vi "SEM shutter.vi"(6 "Shutter close":bool, 7 "delay (ms)":u32=1000, 8 "Shutter AO4":tag="Log/ao3", 9 "Shutter AO3":tag="Log/ao2", 10 "Shutter AO2":tag="Log/ao1", 11 "Shutter AO1":tag="Log/ao0") -> (0 "error out":errorcluster)   [LabVIEW 2018]
uses:
  <vilib>/DAQmx/write.llb/DAQmx Write (Analog 1D DBL NChan 1Samp).vi
  <vilib>/DAQmx/create/channels.llb/DAQmx Create Channel (AO-Voltage-Basic).vi
  <vilib>/DAQmx/miscellaneous.llb/DAQmx Fill In Error Info.vi
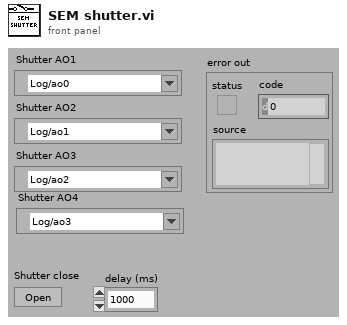
[diagram p1: front panel]
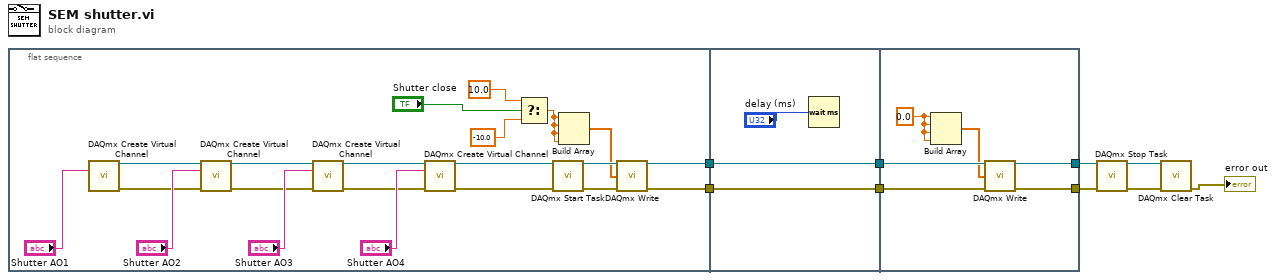
[diagram p0: block diagram]
diagram:
  n1 = flat-sequence {
    tunnel: [w28] -> w4
    tunnel: [w27] -> w2
    tunnel: w4 -> [w33]
    tunnel: [w33] -> w3
    tunnel: w2 -> [w32]
    tunnel: [w32] -> w1
    tunnel: [w36] -> w8
    tunnel: [w38] -> w9
    tunnel: w3 -> [w39]
    tunnel: w1 -> [w37]
    frame #0 {
      n2 = call-poly <vilib>:"DAQmx Create Virtual Channel.vi"("physical channels"="Shutter AO1") -> ("task out"=w20:refnum<k21>, "error out"=w19:errorcluster)  [unwired: 13 in]
      n3 = call-poly <vilib>:"DAQmx Create Virtual Channel.vi"("task in"=w20, "physical channels"="Shutter AO2", "error in"=w19) -> ("task out"=w12:refnum<k21>, "error out"=w11:errorcluster)  [unwired: 11 in]
      n4 = call-poly <vilib>:"DAQmx Create Virtual Channel.vi"("task in"=w12, "physical channels"="Shutter AO3", "error in"=w11) -> ("task out"=w14:refnum<k21>, "error out"=w13:errorcluster)  [unwired: 11 in]
      n5 = call-poly <vilib>:"DAQmx Create Virtual Channel.vi"("task in"=w14, "physical channels"="Shutter AO4", "error in"=w13) -> ("task out"=w16:refnum<k21>, "error out"=w15:errorcluster)  [unwired: 11 in]
      n6 = Select(t=10.0, s="Shutter close", f=-10.0) -> (s? t:f=w10:dbl)
      n7 = call <vilib>:"DAQmx Start Task.vi"("task/channels in"=w16, "error in"=w15) -> ("task out"=w30:refnum<k21>, "error out"=w29:errorcluster)  [unwired: 12 in]
      n8 = Build Array(w10, w10, w10, w10) -> (w22:dbl[])
      n9 = call-poly <vilib>:"DAQmx Write.vi"("task/channels in"=w30, "data"=w22, "error in"=w29) -> ("task out"=w28:refnum<k21>, "error out"=w27:errorcluster)  [unwired: 10 in, 1 out]
    }
    frame #1 {
      n10 = Wait (ms)(milliseconds to wait="delay (ms)") -> ()  [unwired: 1 out]
    }
    frame #2 {
      w34 = 0.0 ("element")
      n11 = Build Array(w34, w34, w34, w34) -> (w35:dbl[])
      n12 = call-poly <vilib>:"DAQmx Write.vi"("task/channels in"=w39, "data"=w35, "error in"=w37) -> ("task out"=w38:refnum<k21>, "error out"=w36:errorcluster)  [unwired: 10 in, 1 out]
    }
  }
  n13 = call <vilib>:"DAQmx Stop Task.vi"("task/channels in"=w9, "error in"=w8) -> ("task out"=w6:refnum<k21>, "error out"=w7:errorcluster)  [unwired: 12 in]
  n14 = call <vilib>:"DAQmx Clear Task.vi"("task in"=w6, "error in"=w7) -> ("error out"=→"error out":errorcluster)  [unwired: 13 in]
